vi "TDD一致性.vi"(0 "TDD filePath":path caption="TDD file Path", 1 "Mating Upper Spec":dbl, 2 "Mating Lower Spec":dbl, 3 "Cable Upper Spec":dbl, 4 "Cable Lower Spec":dbl, 5 "MatingPer":dbl, 6 "CablePer":dbl, 7 "Mating标准差规格":dbl, 8 "Mating Area":dbl, 9 "Cable标准差规格":dbl, 10 "Cable Area":dbl, 11 "Dialog":bool) -> (14 "结果":T1, 15 "测试信息":string)   [LabVIEW 2011]
uses:
  <vilib>/Utility/file.llb/Read From Spreadsheet File (DBL).vi
  <vilib>/Analysis/NI_AALBase.lvlib
panel:
  out "最大最小值规格":T2
  out "最大最小值判定":T3
  out "最大最小值":T4
  out "标准差规格值":cluster{"Mating标准差规格":dbl, "Cable标准差规格":dbl}
  in  "标准差规格":cluster{"Mating标准差规格":dbl, "Cable标准差规格":dbl}
  out "标准差判定":T5
  in  "标准差判定":T5
  out "标准差值":T6
  in  "标准差":T6 {"Cable最小值标准差" format="%0.2f"; "Cable最大值标准差" format="%0.2f"; "Mating最小标注差" format="%0.2f"; "Mating最大标准差" format="%0.2f"}
  out "Cable最小值标准差判定":bool
  out "Cable最大值标准差判定":bool
  out "Mating最小值标准差判定":bool
  out "Mating最大值标准差判定":bool
  out "Cable最小值判定":bool
  out "Cable最大值判定":bool
  out "Mating最小值判定":bool
  out "Mating最大值判定":bool
  out "CableLowerValue":dbl
  out "CableUpperValue":dbl
  out "MatingLowerValue":dbl
  out "MatingUpperValue":dbl
  out "Cable最小值":dbl
  out "Cable最大值":dbl
  out "Mating最小值":dbl
  out "Mating最大值":dbl
  out "Cable最小值标准差":dbl format="%0.2f"
  out "Cable最大值标准差":dbl format="%0.2f"
  out "Mating最小标注差":dbl caption="Mating最小值标注差" format="%0.2f"
  out "Mating最大标准差":dbl caption="Mating最大值标准差" format="%0.2f"
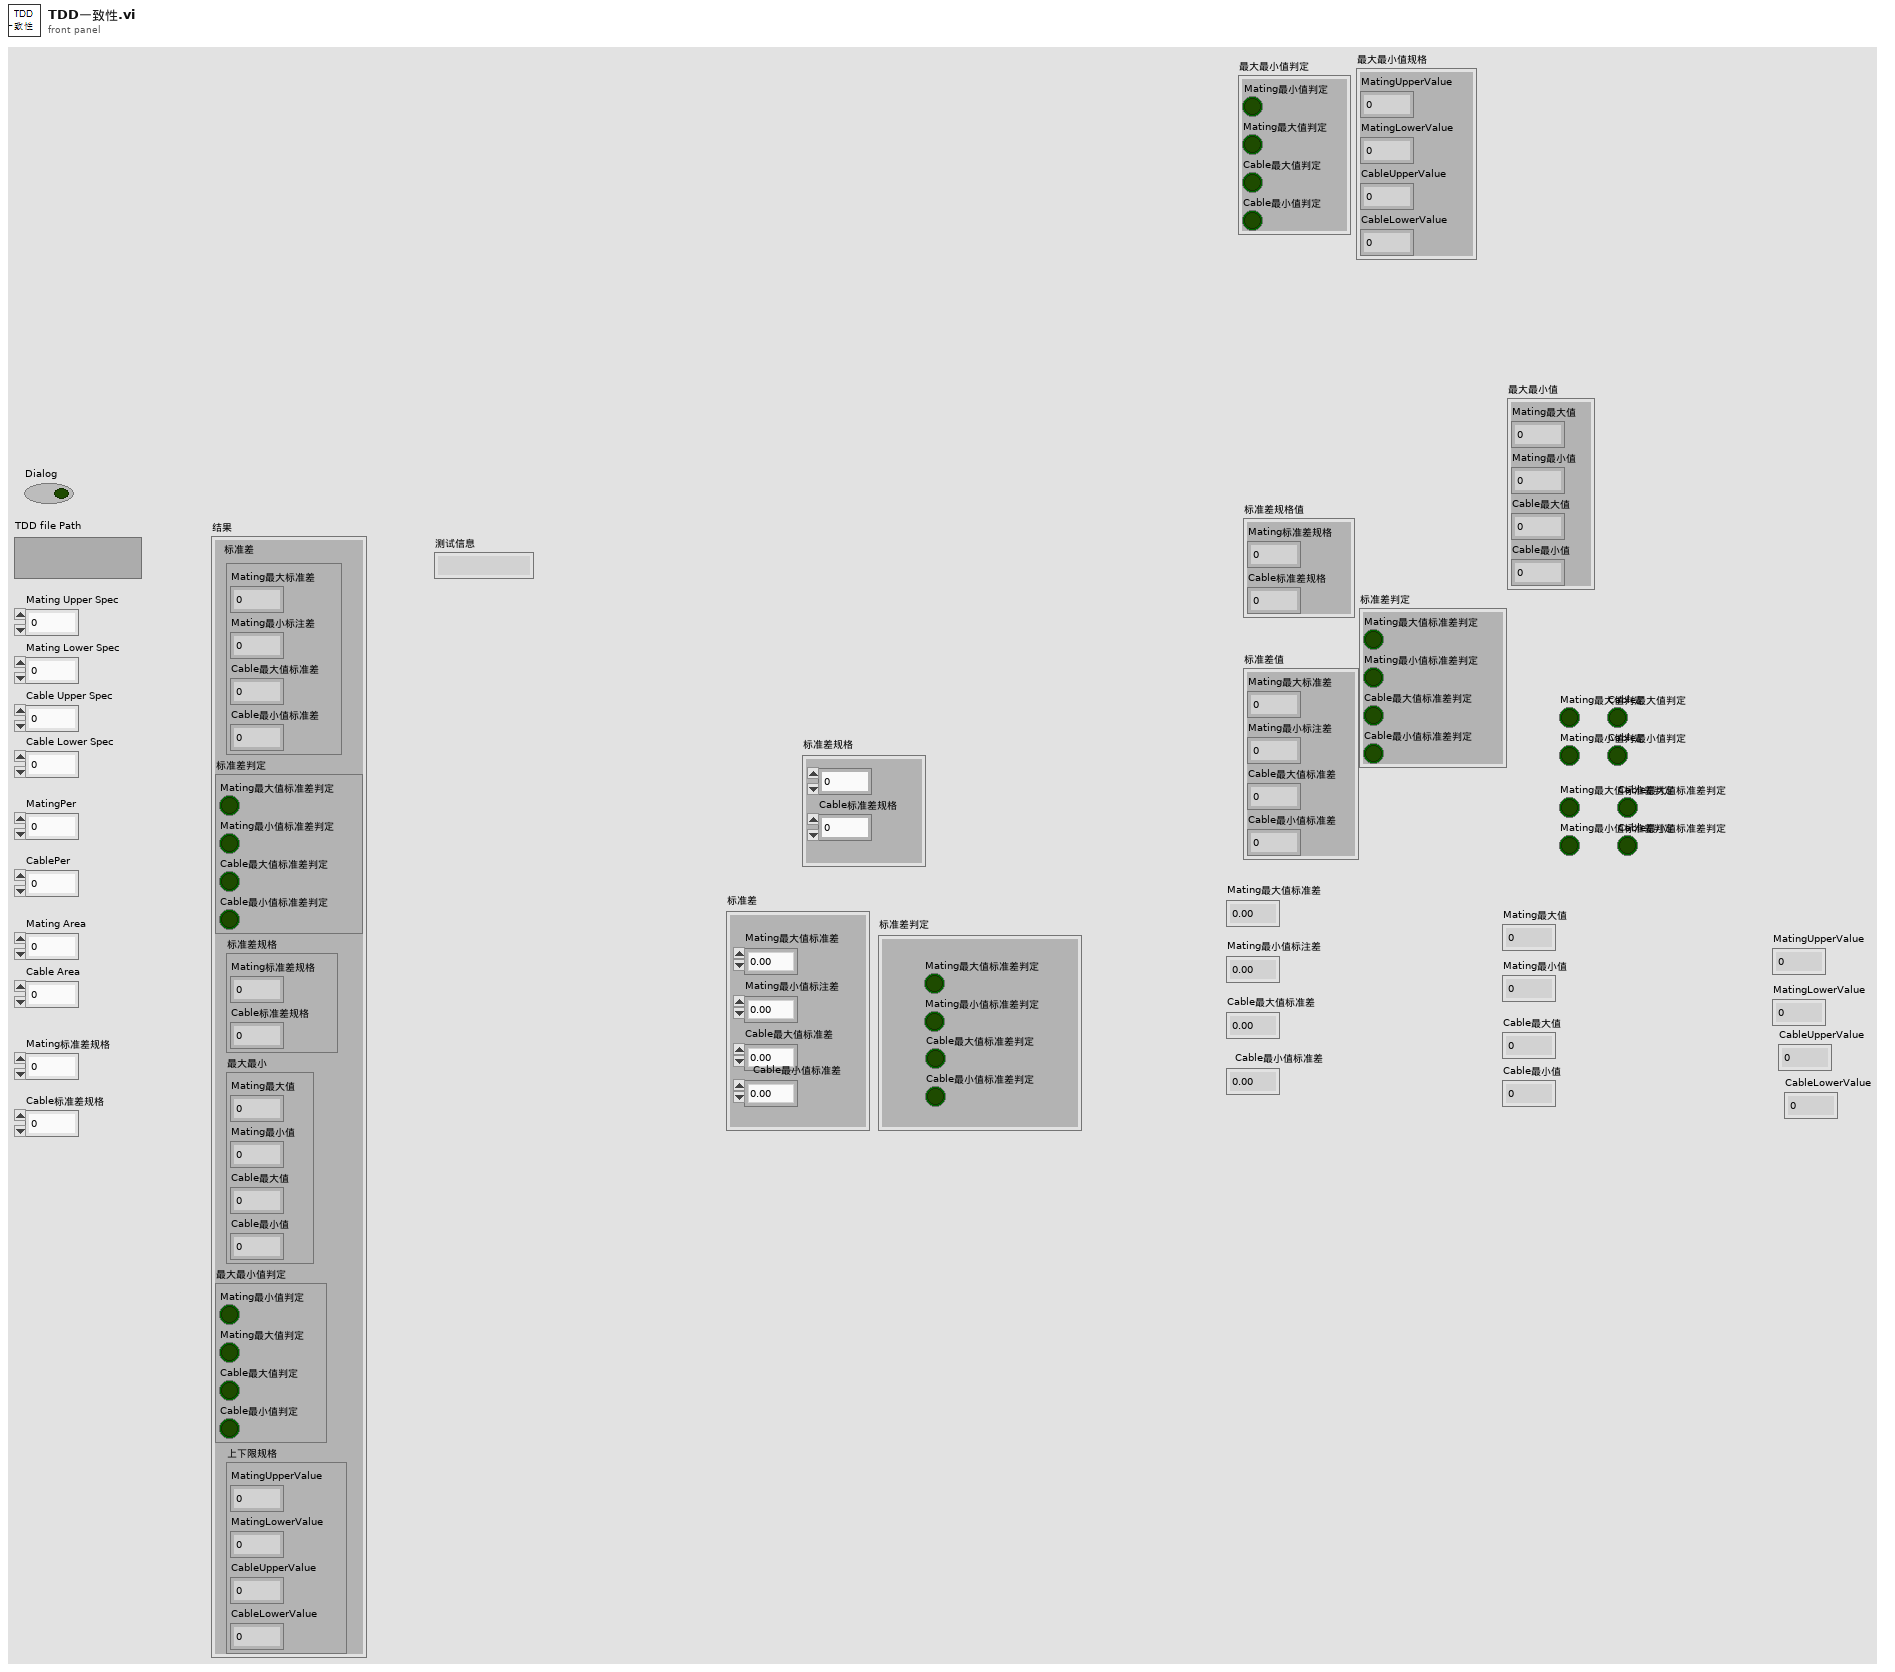
[diagram p1: front panel]
types:
  T1 = cluster{"标准差":cluster{"Mating最大标准差":dbl, "Mating最小标注差":dbl, "Cable最大值标准差":dbl, "Cable最小值标准差":dbl}, "标准差判定":cluster{"Mating最大值标准差判定":bool, "Mating最小值标准差判定":bool, "Cable最大值标准差判定":bool, "Cable最小值标准差判定":bool}, "标准差规格":cluster{"Mating标准差规格":dbl, "Cable标准差规格":dbl}, "最大最小":cluster{"Mating最大值":dbl, "Mating最小值":dbl, "Cable最大值":dbl, "Cable最小值":dbl}, "最大最小值判定":cluster{"Mating最小值判定":bool, "Mating最大值判定":bool, "Cable最大值判定":bool, "Cable最小值判定":bool}, "上下限规格":cluster{"MatingUpperValue":dbl, "MatingLowerValue":dbl, "CableUpperValue":dbl, "CableLowerValue":dbl}}
  T2 = cluster{"MatingUpperValue":dbl, "MatingLowerValue":dbl, "CableUpperValue":dbl, "CableLowerValue":dbl}
  T3 = cluster{"Mating最小值判定":bool, "Mating最大值判定":bool, "Cable最大值判定":bool, "Cable最小值判定":bool}
  T4 = cluster{"Mating最大值":dbl, "Mating最小值":dbl, "Cable最大值":dbl, "Cable最小值":dbl}
  T5 = cluster{"Mating最大值标准差判定":bool, "Mating最小值标准差判定":bool, "Cable最大值标准差判定":bool, "Cable最小值标准差判定":bool}
  T6 = cluster{"Mating最大标准差":dbl, "Mating最小标注差":dbl, "Cable最大值标准差":dbl, "Cable最小值标准差":dbl}
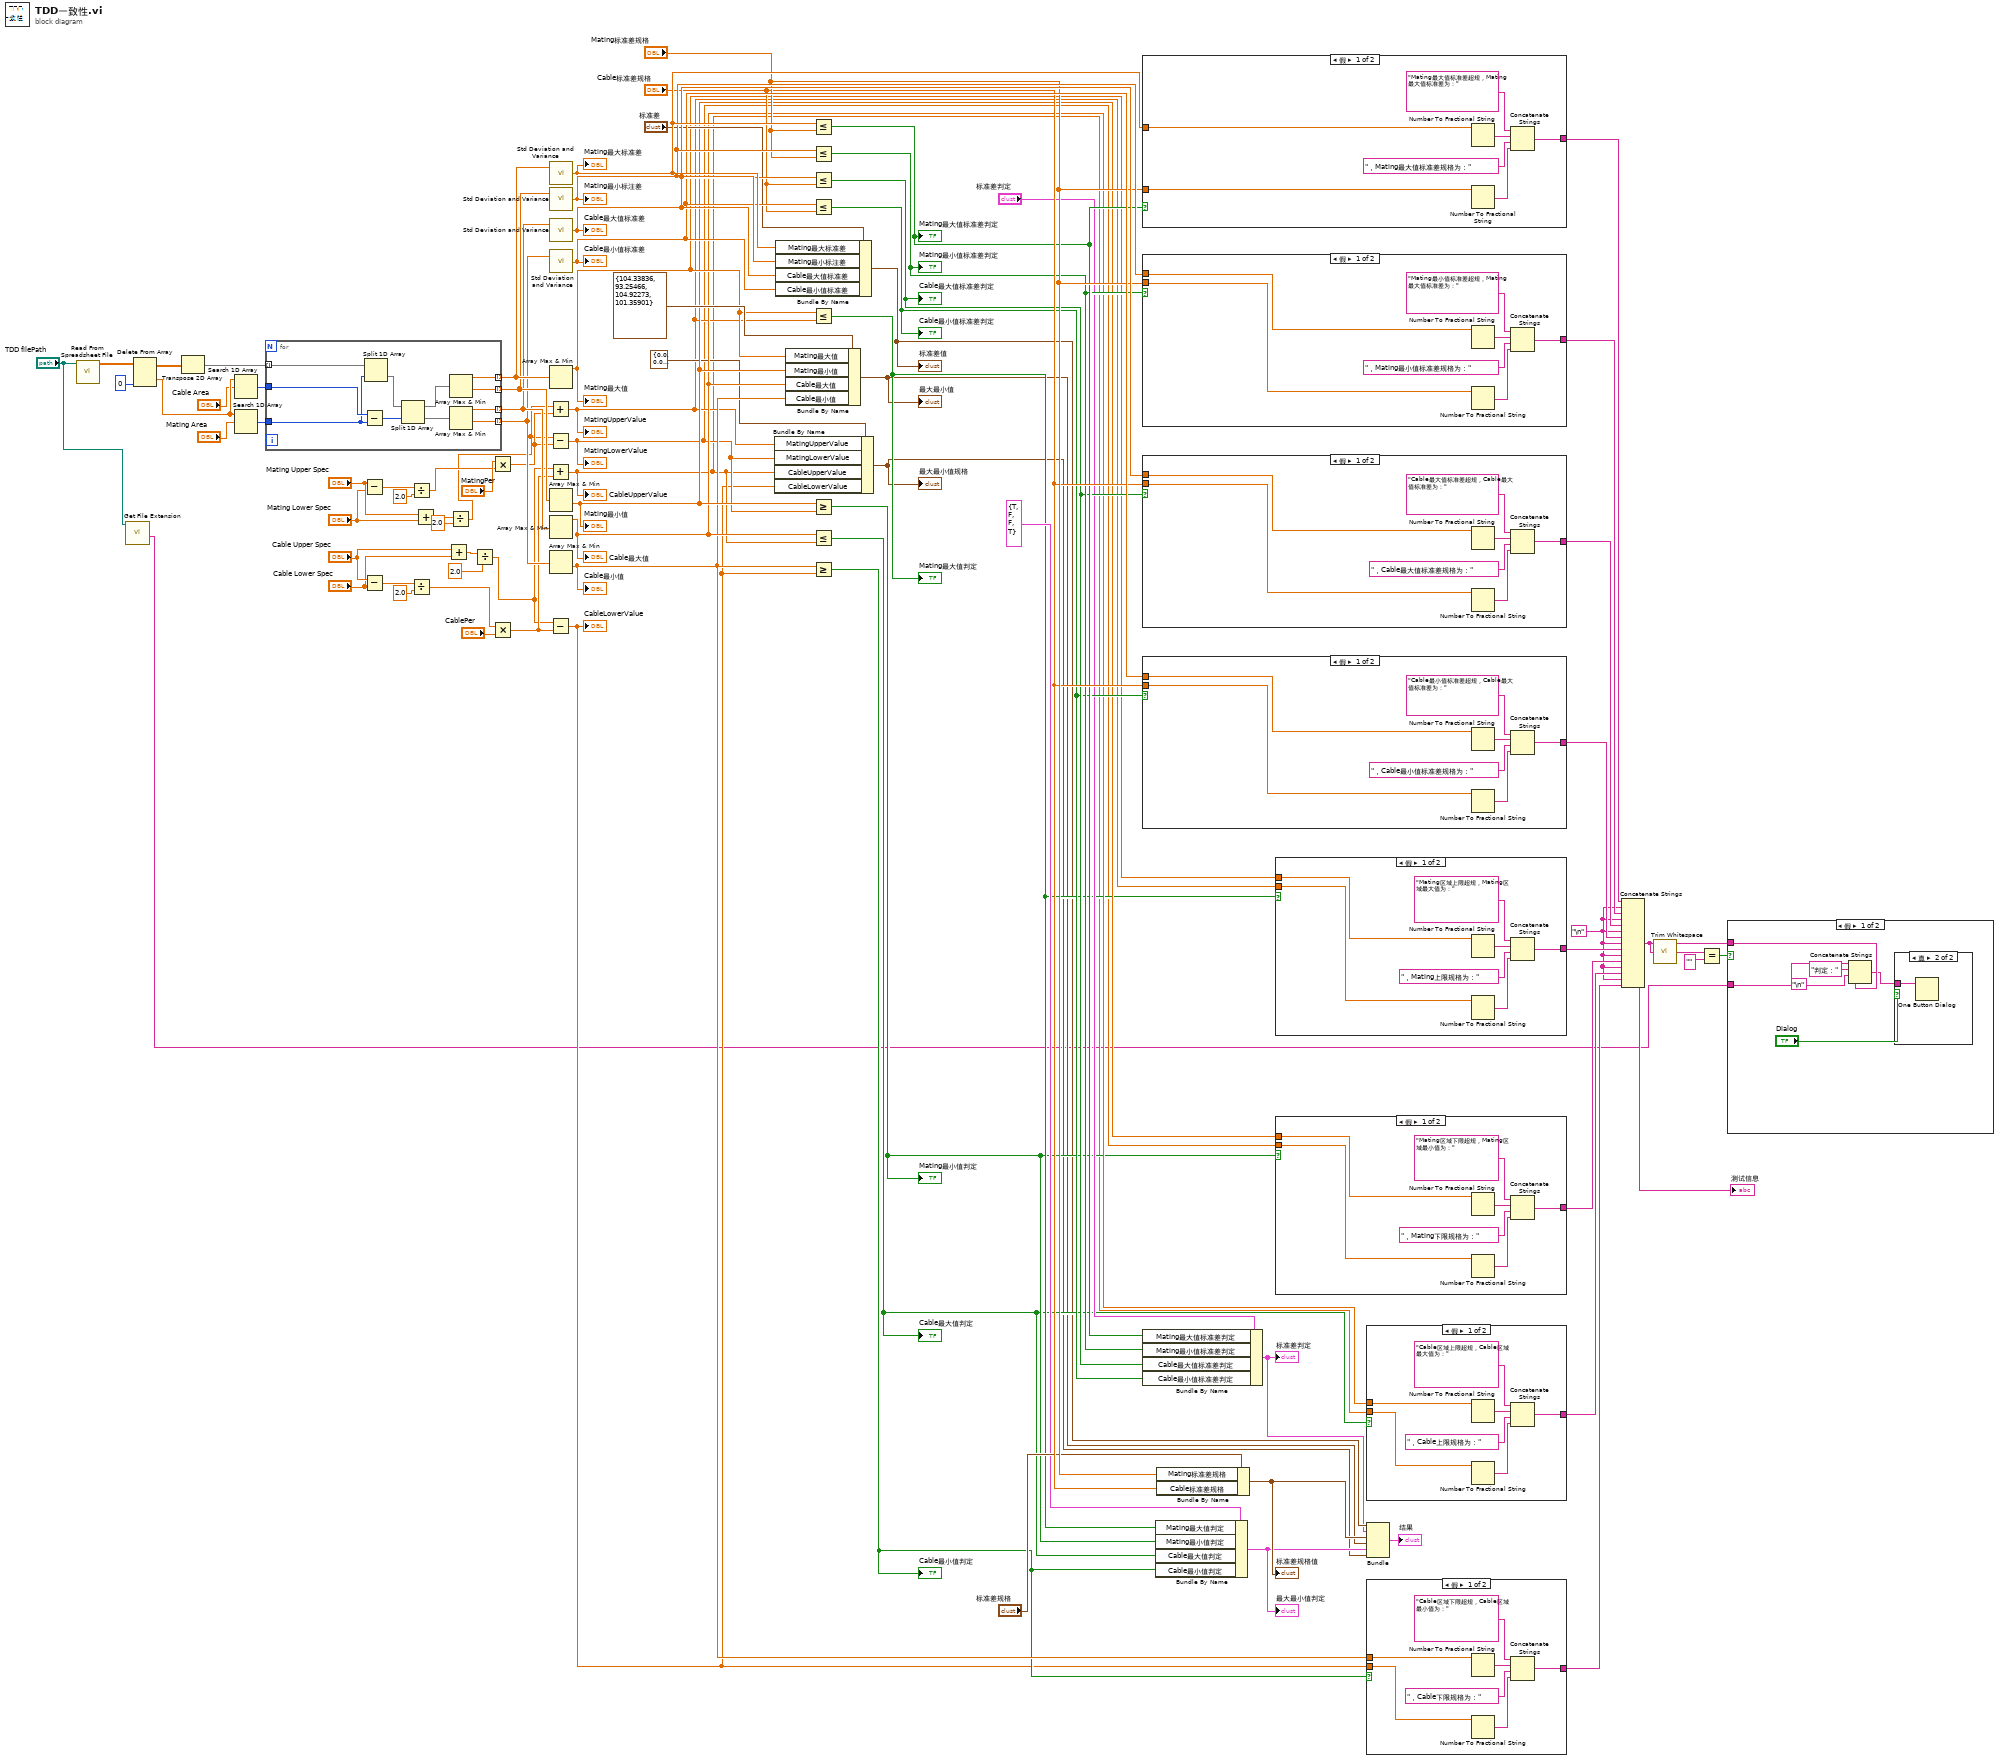
[diagram p0: block diagram]
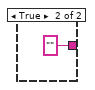
[diagram p4: hidden frame]
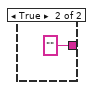
[diagram p5: hidden frame]
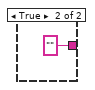
[diagram p6: hidden frame]
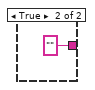
[diagram p7: hidden frame]
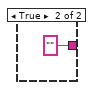
[diagram p8: hidden frame]
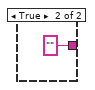
[diagram p9: hidden frame]
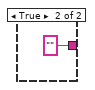
[diagram p10: hidden frame]
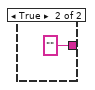
[diagram p11: hidden frame]
diagram:
  w54 = "\n"
  n1 = call-poly <vilib>:"Read From Spreadsheet File.vi"("file path (dialog if empty)"="TDD filePath") -> ("all rows"=w82:dbl[][])  [unwired: 6 in, 4 out]
  n2 = call <vilib>:"Get File Extension.vi"("file"="TDD filePath") -> ("filename without extension"=w1:string)  [unwired: 7 in, 3 out]
  n3 = Delete From Array(array=w82, index (col)=0 ("禁用的索引 (列)")) -> (deleted portion=w80:dbl[], array with subset deleted=w75:dbl[][])  [unwired: 2 in]
  n4 = Transpose 2D Array(2D array=w75) -> (transposed array=w78:dbl[][])
  n5 = Search 1D Array(1D array=w80, element="Cable Area") -> (index of element=w76:i32)  [unwired: 1 in]
  n6 = Search 1D Array(1D array=w80, element="Mating Area") -> (index of element=w77:i32)  [unwired: 1 in]
  n7 = for {
    tunnel: w78 -> [w94] mode=indexing
    tunnel: w77 -> [w92]
    tunnel: w76 -> [w93]
    tunnel: [w88] -> w74 mode=indexing
    tunnel: [w87] -> w73 mode=indexing
    tunnel: [w85] -> w72 mode=indexing
    tunnel: [w84] -> w71 mode=indexing
    n8 = Subtract(x=w93, y=w92) -> (x-y=w90:i32)
    n9 = Split 1D Array(array=w94, index=w92) -> (second subarray=w91:dbl[])  [unwired: 1 out]
    n10 = Split 1D Array(array=w91, index=w90) -> (first subarray=w89:dbl[], second subarray=w86:dbl[])
    n11 = Array Max & Min(array=w89) -> (max value=w88:dbl, min value=w87:dbl)  [unwired: 2 out]
    n12 = Array Max & Min(array=w86) -> (max value=w85:dbl, min value=w84:dbl)  [unwired: 2 out]
  }
  n13 = Subtract(x="Mating Upper Spec", y="Mating Lower Spec") -> (x-y=w70:dbl)
  n14 = Subtract(x="Cable Upper Spec", y="Cable Lower Spec") -> (x-y=w12:dbl)
  n15 = Divide(x=w70, y=2.0) -> (x/y=w67:dbl)
  n16 = Divide(x=w12, y=2.0) -> (x/y=w63:dbl)
  n17 = Add(x="Mating Upper Spec", y="Mating Lower Spec") -> (x+y=w6:dbl)
  n18 = Add(x="Cable Upper Spec", y="Cable Lower Spec") -> (x+y=w11:dbl)
  n19 = Divide(x=w6, y=2.0) -> (x/y=w4:dbl)
  n20 = Divide(x=w11, y=2.0) -> (x/y=w9:dbl)
  n21 = Multiply(x="MatingPer", y=w67) -> (x*y=w66:dbl)
  n22 = Multiply(x=w63, y="CablePer") -> (x*y=w62:dbl)
  n23 = Add(x=w4, y=w66) -> (x+y=w24:dbl)
  "MatingUpperValue" <- w24
  n24 = Subtract(x=w4, y=w66) -> (x-y=w23:dbl)
  "MatingLowerValue" <- w23
  n25 = Add(x=w9, y=w62) -> (x+y=w22:dbl)
  "CableUpperValue" <- w22
  n26 = Subtract(x=w9, y=w62) -> (x-y=w21:dbl)
  "CableLowerValue" <- w21
  n27 = call <vilib>:"Std Deviation and Variance.vi"("X"=w74) -> ("standard deviation"=w48:dbl)  [unwired: 1 in, 2 out]
  "Mating最大标准差" <- w48
  n28 = call <vilib>:"Std Deviation and Variance.vi"("X"=w73) -> ("standard deviation"=w47:dbl)  [unwired: 1 in, 2 out]
  "Mating最小标注差" <- w47
  n29 = call <vilib>:"Std Deviation and Variance.vi"("X"=w72) -> ("standard deviation"=w46:dbl)  [unwired: 1 in, 2 out]
  "Cable最大值标准差" <- w46
  n30 = call <vilib>:"Std Deviation and Variance.vi"("X"=w71) -> ("standard deviation"=w45:dbl)  [unwired: 1 in, 2 out]
  "Cable最小值标准差" <- w45
  n31 = Array Max & Min(array=w74) -> (max value=w34:dbl)  [unwired: 3 out]
  "Mating最大值" <- w34
  n32 = Array Max & Min(array=w73) -> (min value=w33:dbl)  [unwired: 3 out]
  "Mating最小值" <- w33
  n33 = Array Max & Min(array=w72) -> (max value=w32:dbl)  [unwired: 3 out]
  "Cable最大值" <- w32
  n34 = Array Max & Min(array=w71) -> (min value=w31:dbl)  [unwired: 3 out]
  "Cable最小值" <- w31
  n35 = Bundle By Name(cluster=T2 {"MatingUpperValue"=0.0, "MatingLowerValue"=0.0, "CableUpperValue"=0.0, "CableLowerValue"=0.0} ("上下限规格"), "MatingUpperValue"=w24, "MatingLowerValue"=w23, "CableUpperValue"=w22, "CableLowerValue"=w21) -> (w15:T2)
  "最大最小值规格" <- w15
  n36 = Bundle By Name(cluster="标准差", "Mating最大标准差"=w48, "Mating最小标注差"=w47, "Cable最大值标准差"=w46, "Cable最小值标准差"=w45) -> (w20:T6)
  "标准差值" <- w20
  n37 = Bundle By Name(cluster=T4 {"Mating最大值"=104.33836, "Mating最小值"=93.25466, "Cable最大值"=104.92273, "Cable最小值"=101.35901} ("最大最小"), "Mating最大值"=w34, "Mating最小值"=w33, "Cable最大值"=w32, "Cable最小值"=w31) -> (w17:T4)
  "最大最小值" <- w17
  n38 = Less Or Equal?(x=w48, y="Mating标准差规格") -> (x <= y?=w42:bool)
  "Mating最大值标准差判定" <- w42
  n39 = Less Or Equal?(x=w47, y="Mating标准差规格") -> (x <= y?=w41:bool)
  "Mating最小值标准差判定" <- w41
  n40 = Less Or Equal?(x=w46, y="Cable标准差规格") -> (x <= y?=w40:bool)
  "Cable最大值标准差判定" <- w40
  n41 = Less Or Equal?(x=w45, y="Cable标准差规格") -> (x <= y?=w39:bool)
  "Cable最小值标准差判定" <- w39
  n42 = Less Or Equal?(x=w34, y=w24) -> (x <= y?=w29:bool)
  "Mating最大值判定" <- w29
  n43 = Greater Or Equal?(x=w33, y=w23) -> (x >= y?=w28:bool)
  "Mating最小值判定" <- w28
  n44 = Less Or Equal?(x=w32, y=w22) -> (x <= y?=w27:bool)
  "Cable最大值判定" <- w27
  n45 = Greater Or Equal?(x=w31, y=w21) -> (x >= y?=w26:bool)
  "Cable最小值判定" <- w26
  n46 = case shown="假" w42 {
    tunnel: [w96 ""] -> w61
    tunnel: w48 -> [w100 _]
    tunnel: "Mating标准差规格" -> [w95 _]
    frame False {
      n47 = Number To Fractional String(number=w100) -> (F-format string=w99:string)  [unwired: 3 in]
      n48 = Number To Fractional String(number=w95) -> (F-format string=w97:string)  [unwired: 3 in]
      n49 = Concatenate Strings("Mating最大值标准差超规，Mating最大值标准差为：", w99, "，Mating最大值标准差规格为：" ("字符串"), w97) -> (w96:string)
    }
    frame True {
    }
  }
  n50 = case shown="假" w41 {
    tunnel: [w105 ""] -> w60
    tunnel: w47 -> [w104 _]
    tunnel: "Mating标准差规格" -> [w103 _]
    frame False {
      n51 = Number To Fractional String(number=w104) -> (F-format string=w108:string)  [unwired: 3 in]
      n52 = Number To Fractional String(number=w103) -> (F-format string=w106:string)  [unwired: 3 in]
      n53 = Concatenate Strings("Mating最小值标准差超规，Mating最大值标准差为：", w108, "，Mating最小值标准差规格为：" ("字符串"), w106) -> (w105:string)
    }
    frame True {
    }
  }
  n54 = case shown="假" w40 {
    tunnel: [w113 ""] -> w59
    tunnel: w46 -> [w112 _]
    tunnel: "Cable标准差规格" -> [w111 _]
    frame False {
      n55 = Number To Fractional String(number=w112) -> (F-format string=w116:string)  [unwired: 3 in]
      n56 = Number To Fractional String(number=w111) -> (F-format string=w114:string)  [unwired: 3 in]
      n57 = Concatenate Strings("Cable最大值标准差超规，Cable最大值标准差为：", w116, "，Cable最大值标准差规格为：" ("字符串"), w114) -> (w113:string)
    }
    frame True {
    }
  }
  n58 = case shown="假" w39 {
    tunnel: [w121 ""] -> w58
    tunnel: w45 -> [w120 _]
    tunnel: "Cable标准差规格" -> [w119 _]
    frame False {
      n59 = Number To Fractional String(number=w120) -> (F-format string=w124:string)  [unwired: 3 in]
      n60 = Number To Fractional String(number=w119) -> (F-format string=w122:string)  [unwired: 3 in]
      n61 = Concatenate Strings("Cable最小值标准差超规，Cable最大值标准差为：", w124, "，Cable最小值标准差规格为：" ("字符串"), w122) -> (w121:string)
    }
    frame True {
    }
  }
  n62 = Bundle By Name(cluster="标准差判定", "Mating最大值标准差判定"=w42, "Mating最小值标准差判定"=w41, "Cable最大值标准差判定"=w40, "Cable最小值标准差判定"=w39) -> (w19:T5)
  "标准差判定" <- w19
  n63 = Bundle By Name(cluster=T3 {"Mating最小值判定"=TRUE, "Mating最大值判定"=FALSE, "Cable最大值判定"=FALSE, "Cable最小值判定"=TRUE} ("最大最小值判定"), "Mating最大值判定"=w29, "Mating最小值判定"=w28, "Cable最大值判定"=w27, "Cable最小值判定"=w26) -> (w16:T3)
  "最大最小值判定" <- w16
  n64 = Bundle By Name(cluster="标准差规格", "Mating标准差规格"="Mating标准差规格", "Cable标准差规格"="Cable标准差规格") -> (w18:cluster{"Mating标准差规格":dbl, "Cable标准差规格":dbl})
  "标准差规格值" <- w18
  n65 = case shown="假" w29 {
    tunnel: [w130 ""] -> w57
    tunnel: w34 -> [w133 _]
    tunnel: w24 -> [w128 _]
    frame False {
      n66 = Number To Fractional String(number=w133) -> (F-format string=w131:string)  [unwired: 3 in]
      n67 = Number To Fractional String(number=w128) -> (F-format string=w127:string)  [unwired: 3 in]
      n68 = Concatenate Strings("Mating区域上限超规，Mating区域最大值为：", w131, "，Mating上限规格为：" ("字符串"), w127) -> (w130:string)
    }
    frame True {
    }
  }
  n69 = case shown="假" w28 {
    tunnel: [w137 ""] -> w56
    tunnel: w33 -> [w136 _]
    tunnel: w23 -> [w135 _]
    frame False {
      n70 = Number To Fractional String(number=w136) -> (F-format string=w140:string)  [unwired: 3 in]
      n71 = Number To Fractional String(number=w135) -> (F-format string=w138:string)  [unwired: 3 in]
      n72 = Concatenate Strings("Mating区域下限超规，Mating区域最小值为：", w140, "，Mating下限规格为：" ("字符串"), w138) -> (w137:string)
    }
    frame True {
    }
  }
  n73 = case shown="假" w27 {
    tunnel: [w145 ""] -> w55
    tunnel: w32 -> [w144 _]
    tunnel: w22 -> [w143 _]
    frame False {
      n74 = Number To Fractional String(number=w144) -> (F-format string=w148:string)  [unwired: 3 in]
      n75 = Number To Fractional String(number=w143) -> (F-format string=w146:string)  [unwired: 3 in]
      n76 = Concatenate Strings("Cable区域上限超规，Cable区域最大值为：", w148, "，Cable上限规格为：" ("字符串"), w146) -> (w145:string)
    }
    frame True {
    }
  }
  n77 = Bundle("标准差"=w20, "标准差判定"=w19, "标准差规格"=w18, "最大最小"=w17, "最大最小值判定"=w16, "上下限规格"=w15) -> (→"结果":T1)  [unwired: 1 in]
  n78 = case shown="假" w26 {
    tunnel: [w153 ""] -> w53
    tunnel: w31 -> [w152 _]
    tunnel: w21 -> [w151 _]
    frame False {
      n79 = Number To Fractional String(number=w152) -> (F-format string=w156:string)  [unwired: 3 in]
      n80 = Number To Fractional String(number=w151) -> (F-format string=w154:string)  [unwired: 3 in]
      n81 = Concatenate Strings("Cable区域下限超规，Cable区域最小值为：", w156, "，Cable下限规格为：" ("字符串"), w154) -> (w153:string)
    }
    frame True {
    }
  }
  n82 = Concatenate Strings(w61, w54, w60, w54, w59, w54, w58, w54, w57, w54, w56, w54, w55, w54, w53) -> (w49:string)
  "测试信息" <- w49
  n83 = call <vilib>:"Trim Whitespace.vi"("string"=w49) -> ("trimmed string"=w52:string)  [unwired: 1 in]
  n84 = Equal?(x=w52, y="") -> (x = y?=w50:bool)
  n85 = case shown="假" w50 {
    tunnel: w49 -> [w161 _]
    tunnel: w1 -> [w164 _]
    frame False {
      n86 = Concatenate Strings(w164, "判定：" ("字符串"), "\n", w161) -> (w160:string)
      n87 = case shown="真" "Dialog" {
        tunnel: w160 -> [_ w165]
        frame False {
        }
        frame True {
          n88 = One Button Dialog(message=w165) -> ()  [unwired: 1 in, 1 out]
        }
      }
    }
    frame True {
    }
  }
